vi "VS-Acquire One Channel.vi"(1 "maximum value":dbl=5.0, 2 "minimum value":dbl=-5.0, 3 "input terminal configuration":i32(ring)=-1 items=["default"=-1, "RSE"=10083, "NRSE"=10078, "Differential"=10106, "Pseudodifferential"=12529], 7 "index":i32, 11 "error in":errorcluster) -> (8 "mean":dbl format="%0.2f", 15 "error out":errorcluster)   [LabVIEW 2020]
uses:
  <vilib>/DAQmx/read.llb/DAQmx Read (Analog 1D DBL 1Chan NSamp).vi
  <vilib>/Analysis/baseanly.llb/Mean (DBL).vi
  <vilib>/DAQmx/create/channels.llb/DAQmx Create Channel (AI-Voltage-Basic).vi
  <vilib>/DAQmx/configure/timing.llb/DAQmx Timing (Sample Clock).vi
  <vilib>/DAQmx/miscellaneous.llb/DAQmx Fill In Error Info.vi
  <vilib>/Analysis/NI_AALBase.lvlib
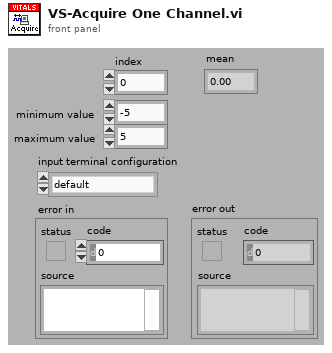
[diagram p1: front panel]
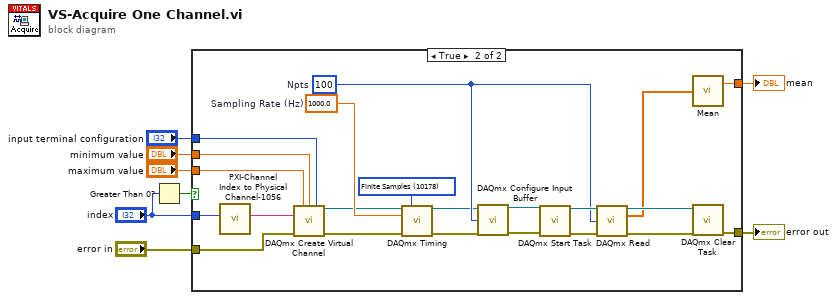
[diagram p0: block diagram]
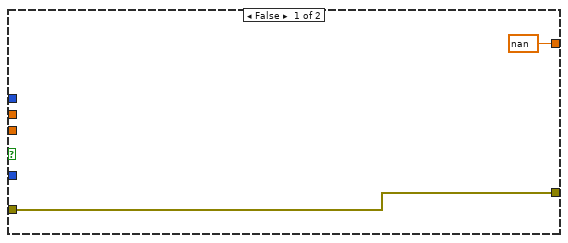
[diagram p2: hidden frame]
diagram:
  n1 = Greater Than 0?(x="index") -> (x > 0?=w5:bool)
  n2 = case shown="True" w5 {
    tunnel: "index" -> [_ w18]
    tunnel: [nan ("mean") w17] -> w8
    tunnel: [w10 w16] -> w7
    tunnel: "error in" -> [w10 w15]
    tunnel: "maximum value" -> [_ w14]
    tunnel: "minimum value" -> [_ w13]
    tunnel: "input terminal configuration" -> [_ w12]
    frame False {
    }
    frame True {
      w25 = 1000.0  # Sampling Rate (Hz)
      w26 = u32 100  # Npts
      w32 = 10178 items=["Finite Samples"=10178, "Continuous Samples"=10123, "Hardware Timed Single Point"=12522] ("sample mode")
      n3 = call "PXI-Channel Index to Physical Channel-1056.vi"("index"=w18) -> ("element"=w19:tag)  [unwired: 10 in]
      n4 = call-poly <vilib>:"DAQmx Create Virtual Channel.vi"("maximum value"=w14, "minimum value"=w13, "input terminal configuration"=w12, "physical channels"=w19, "error in"=w15) -> ("task out"=w11:refnum<k21>, "error out"=w24:errorcluster)  [unwired: 9 in]
      n5 = call-poly <vilib>:"DAQmx Timing.vi"("task/channels in"=w11, "sample mode"=w32, "rate"=w25, "error in"=w24) -> ("task out"=w21:refnum<k21>, "error out"=w23:errorcluster)  [unwired: 10 in]
      n6 = call <vilib>:"DAQmx Configure Input Buffer.vi"("task/channels in"=w21, "buffer size (in samples per channel)"=w26, "error in"=w23) -> ("task out"=w20:refnum<k21>, "error out"=w22:errorcluster)  [unwired: 11 in]
      n7 = call <vilib>:"DAQmx Start Task.vi"("task/channels in"=w20, "error in"=w22) -> ("task out"=w27:refnum<k21>, "error out"=w28:errorcluster)  [unwired: 12 in]
      n8 = call-poly <vilib>:"DAQmx Read.vi"("task/channels in"=w27, "number of samples per channel"=w26, "error in"=w28) -> ("task out"=w30:refnum<k21>, "data"=w29:dbl[], "error out"=w31:errorcluster)  [unwired: 10 in]
      n9 = call-poly <vilib>:"Mean.vi"("X"=w29) -> ("mean"=w17:dbl)  [unwired: 1 out]
      n10 = call <vilib>:"DAQmx Clear Task.vi"("task in"=w30, "error in"=w31) -> ("error out"=w16:errorcluster)  [unwired: 13 in]
    }
  }
  "mean" <- w8
  "error out" <- w7
